vi "VerifyAddress.vi"(8 "error in":errorcluster, 10 "Address(From Response)":u32, 11 "Address #":u8) -> (0 "error out":errorcluster)   [LabVIEW 2020, in "driver_flodx_rtd.lvlib"]
uses:
  <instrlib>/RxnRover/FloDx RTD Driver/driver_flodx_rtd.lvlib
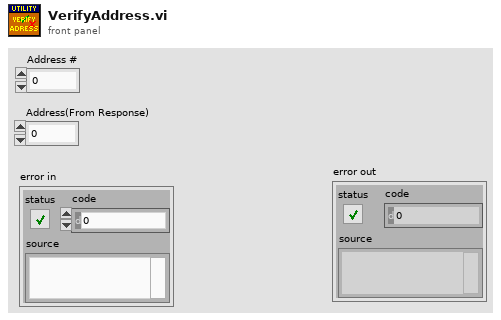
[diagram p1: front panel]
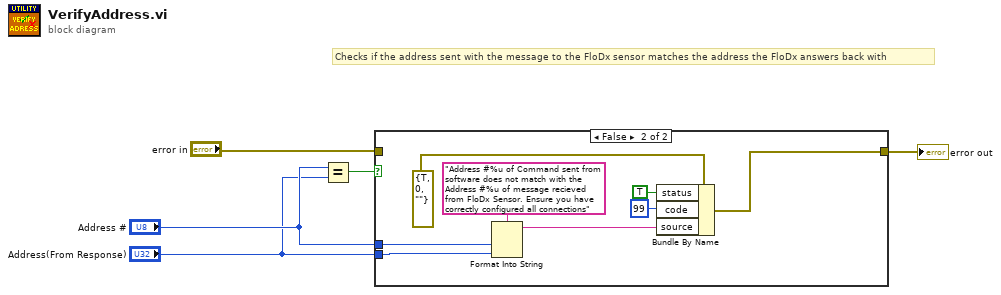
[diagram p0: block diagram]
diagram:
  # "Checks if the address sent with the message to the FloDx sensor matches the address the FloDx answers back with"
  n1 = Equal?(x="Address #", y="Address(From Response)") -> (x = y?=w4:bool)
  n2 = case shown="False" w4 {
    tunnel: [w6 w13] -> w2
    tunnel: "error in" -> [w6 _]
    tunnel: "Address #" -> [_ w8]
    tunnel: "Address(From Response)" -> [_ w7]
    frame True {
    }
    frame False {
      n3 = Format Into String(format string="Address #%u of Command sent from software does not match with the Address #%u of message recieved from FloDx Sensor. Ensure you have correctly configured all connections", w8, w7) -> (resulting string=w9:string)  [unwired: 2 in, 1 out]
      n4 = Bundle By Name(cluster=errorcluster {"status"=TRUE, "code"=0, "source"=""} ("error IO"), "status"=TRUE, "code"=99, "source"=w9) -> (w13:errorcluster)
    }
  }
  "error out" <- w2
